vi "save.vi"(8 "error in (no error)":errorcluster, 9 "base name":string, 10 "folder path":path, 11 "DL090215DataCollection in":refnum<class "DataCollectionDL090215.lvclass">) -> (0 "error out":errorcluster, 3 "DL090215DataCollection out":refnum<class "DataCollectionDL090215.lvclass">)   [LabVIEW 2010, in "DataCollectionDL090215.lvclass"]
uses:
  DataCollectionDL090215.lvclass
  DataCollectionDL090215.lvclass/DataCollectionDL090215.ctl
  DataCollectionDL091104Scaffold/DataCollectionDL091104Scaffold/DataCollectionDL091104Scaffold.lvclass
  common/classes/ErrorController/ErrorController/class_data.vi
  common/classes/ErrorController/ErrorController/ErrorController.lvclass
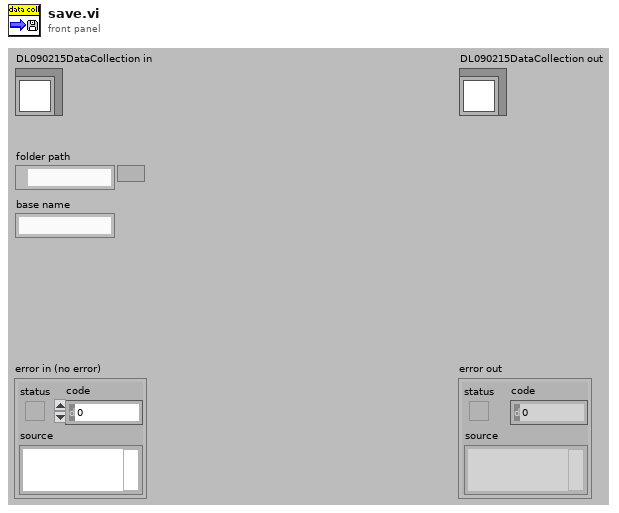
[diagram p1: front panel]
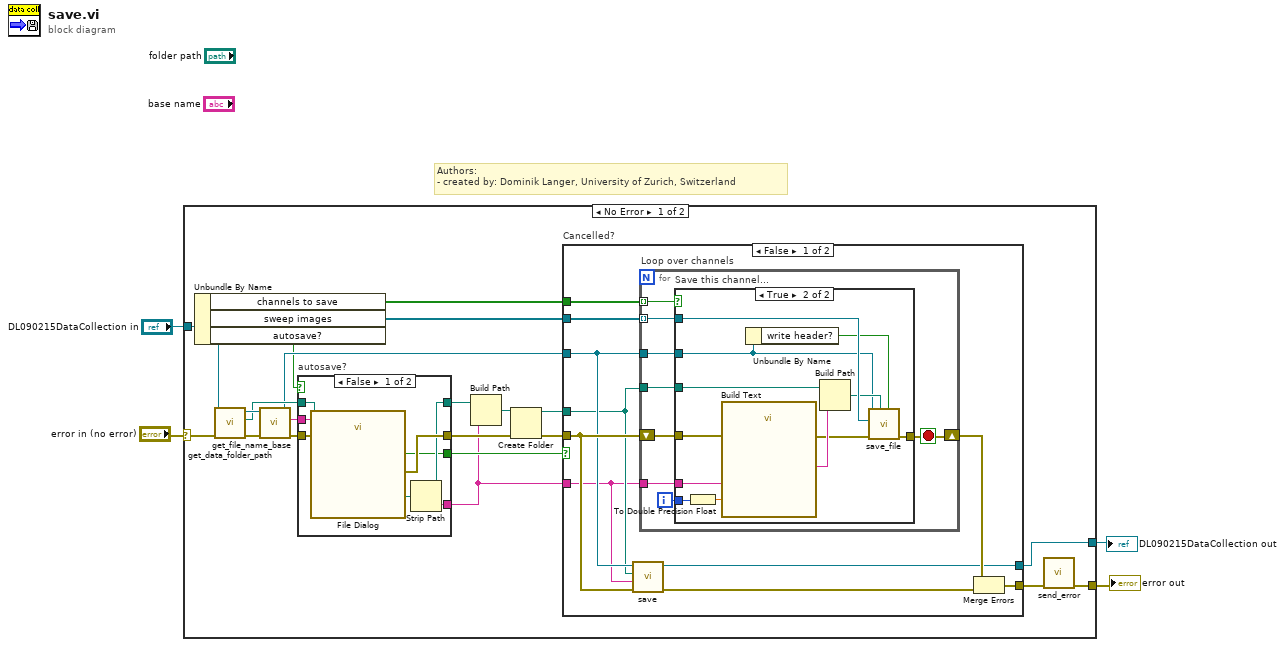
[diagram p0: block diagram]
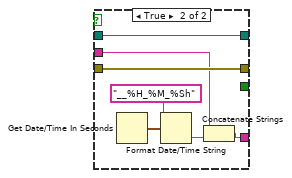
[diagram p4: hidden frame]
diagram:
  # "Authors: \n- created by: Dominik Langer, University of Zurich, Switzerland"
  n1 = case shown="No Error" "error in (no error)" {
    selector: "error in (no error)" -> [w10 w75]
    tunnel: [w18 w75] -> w1
    tunnel: [w11 w74] -> w3
    tunnel: "DL090215DataCollection in" -> [w8 w74]
    frame No Error {
      n2 = Unbundle By Name(w8) -> ("channels to save"=w6:bool[], "sweep images"=w5:refnum<class "ImageCollection.lvclass">[], "autosave?"=w7:bool)
      n3 = call-dynamic "get_data_folder_path.vi"("error in (no error)"=w10, "GenericComponent in"=w8) -> ("error out"=w24:errorcluster, "data folder path"=w21:path, "GenericComponent out"=w25:refnum<class "DataCollectionDL090215.lvclass">)  [unwired: 7 out]
      n4 = call-dynamic "get_file_name_base.vi"("error in (no error)"=w24, "GenericComponent in"=w25) -> ("error out"=w23:errorcluster, "file name base"=w22:string, "GenericComponent out"=w19:refnum<class "DataCollectionDL090215.lvclass">)  [unwired: 7 out]
      n5 = case "autosave?" shown="False" w7 {
        tunnel: w23 -> [w66 w73]
        tunnel: [w65 w73] -> w16
        tunnel: w22 -> [w59 w69]
        tunnel: [w64 w67] -> w12
        tunnel: w21 -> [w61 w72]
        tunnel: [w62 w72] -> w14
        tunnel: [w60 _] -> w20
        frame False {
          n6 = call "File Dialog"("start path"=w61, "default name"=w59, "error in"=w66) -> ("selected path"=w63:path, "cancelled"=w60:bool, "error out"=w65:errorcluster)  [unwired: 4 in, 6 out]
          n7 = Strip Path(path=w63) -> (stripped path=w62:path, name=w64:string)
        }
        frame True {
          n8 = Get Date/Time In Seconds() -> (seconds since 1Jan1904=w70:timestamp)
          n9 = Format Date/Time String(time format string (%c)="__%H_%M_%Sh", seconds (now)=w70) -> (date/time string=w68:string)  [unwired: 1 out]
          n10 = Concatenate Strings(w69, w68) -> (w67:string)
        }
      }
      n11 = Build Path(base path=w14, name or relative path=w12) -> (appended path=w13:path)
      n12 = Create Folder(path (use dialog)=w13, error in=w16) -> (created path=w15:path, error out=w17:errorcluster)  [unwired: 1 in, 1 out]
      n13 = case "Cancelled?" shown="False" w20 {
        tunnel: w5 -> [w33 _]
        tunnel: w17 -> [w31 w58]
        tunnel: w12 -> [w27 _]
        tunnel: w15 -> [w28 _]
        tunnel: [w29 w57] -> w11
        tunnel: [w34 w58] -> w9
        tunnel: w19 -> [w30 w57]
        tunnel: w6 -> [w26 _]
        frame False {
          n14 = call-parent "save.vi"("error in (no error)"=w31, "base name"=w27, "folder path"=w28, "DL090215DataCollection in"=w30) -> ("error out"=w32:errorcluster, "DL090215DataCollection out"=w29:refnum<class "DataCollectionDL090215.lvclass">)  [unwired: 6 in]
          n15 = for "Loop over channels" {
            tunnel: w33 -> [w39] mode=indexing
            tunnel: w27 -> [w41]
            tunnel: w28 -> [w40]
            tunnel: w30 -> [w38]
            shift-right: [w37] -> w35
            shift-left: w31 -> [w43]
            tunnel: w26 -> [w36] mode=indexing
            i -> [w42]
            stop <- w37 stop-if-true
            n16 = case "Save this channel..." shown="True" w36 {
              tunnel: w43 -> [w44 w56]
              tunnel: w42 -> [_ w55]
              tunnel: w41 -> [_ w52]
              tunnel: w40 -> [_ w51]
              tunnel: w39 -> [_ w49]
              tunnel: w38 -> [_ w47]
              tunnel: [w44 w45] -> w37
              frame False {
              }
              frame True {
                n17 = To Double Precision Float(number=w55) -> (double precision float=w53:dbl)
                n18 = call "Build Text"("base"=w52, "channel"=w53, "error in (no error)"=w56) -> ("Result"=w54:string, "error out"=w50:errorcluster)  [unwired: 2 in, 9 out]
                n19 = Unbundle By Name(w47) -> ("write header?"=w46:bool)
                n20 = Build Path(base path=w51, name or relative path=w54) -> (appended path=w48:path)
                n21 = call "save_file.vi"("write header?"=w46, "path"=w48, "error in (no error)"=w50, "ImageCollection in"=w49, "DataCollectionDL090215 in"=w47) -> ("error out"=w45:errorcluster)  [unwired: 5 in, 1 out]
              }
            }
          }
          n22 = Merge Errors(w35, w32) -> (w34:errorcluster)
        }
        frame True {
        }
      }
      n23 = call "send_error.vi"("error in (no error)"=w9) -> ("error out"=w18:errorcluster)  [unwired: 10 in]
    }
    frame Error {
    }
  }
  "error out" <- w1
  "DL090215DataCollection out" <- w3
